vi "Cycle 9 Speed Monitor.vi"(0 "GEA2 Reference In":refnum<k24>, 5 "GEA Inputs":T1={"Source"=228, "Destination"=35} {"Destination" format="%.0x"; "Source" format="%.0x"}, 7 "Standalone?":bool, 11 "Error In":errorcluster) -> (4 "GEA2 Reference Out":refnum<k24>, 6 "Pass/Fail?":bool, 8 "Report Text":string, 15 "Error Out":errorcluster)   [LabVIEW 2016, in "Centauro.lvlib"]
uses:
  Projects/Centauro.lvlib
  Q:/Common/DLLs/GEA3/GeaCommunication.dll
  Common/DLLs/GEA3/GeaCommunication.dll
  Common/LabVIEW GEA2 Toolkit/LabVIEW_GEA2_Toolkit.lvlibp/type defs/Source_Destination.ctl
  Common/LabVIEW GEA2 Toolkit/LabVIEW_GEA2_Toolkit.lvlibp/type defs/ERD Read Data In.ctl
  Common/LabVIEW GEA2 Toolkit/LabVIEW_GEA2_Toolkit.lvlibp/type defs/Data Type.ctl
  Valew Common/type defs/Drive Cycle Engine Request State.ctl
  Common/LabVIEW GEA2 Toolkit/LabVIEW_GEA2_Toolkit.lvlibp
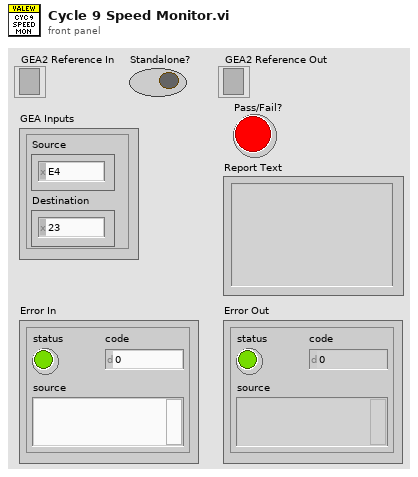
[diagram p1: front panel]
types:
  T1 = typedef "LabVIEW_GEA2_Toolkit.lvlibp/Source_Destination.ctl" = cluster{"Source":u8, "Destination":u8}
  T2 = typedef "LabVIEW_GEA2_Toolkit.lvlibp/ERD Read Data In.ctl" = cluster{"ERD Number":u16, "Data Type":T3}
  T3 = typedef "LabVIEW_GEA2_Toolkit.lvlibp/Data Type.ctl" = enum16{"string", "boolean", "uint8_t", "uint16_t", "uint32_t", "uint64_t", "int8_t", "int16_t", "int32_t", "int64_t"}
  T4 = enum16{"EQ (==)", "NE (!=)", "GT (>)", "LT (<)", "GE (>=)", "LE (<=)", "GTLT(> <)", "GELE (>= <=)", "GELT (>= <)", "GTLE (> <=)", "LTGT (< >)", "LEGE (<= >=)", "LEGT (<= >)", "LTGE (< >=)", "No Comparison"}
  T5 = typedef "Centauro.lvlib/Drive Cycle Engine Request State.ctl" = enum16{"Start", "Stop", "Pause", "Resume", "Select"}
  T6 = typedef "LabVIEW_GEA2_Toolkit.lvlibp/ERD Read Data Out.ctl" = cluster{"ERD Number":u16, "Data":string}
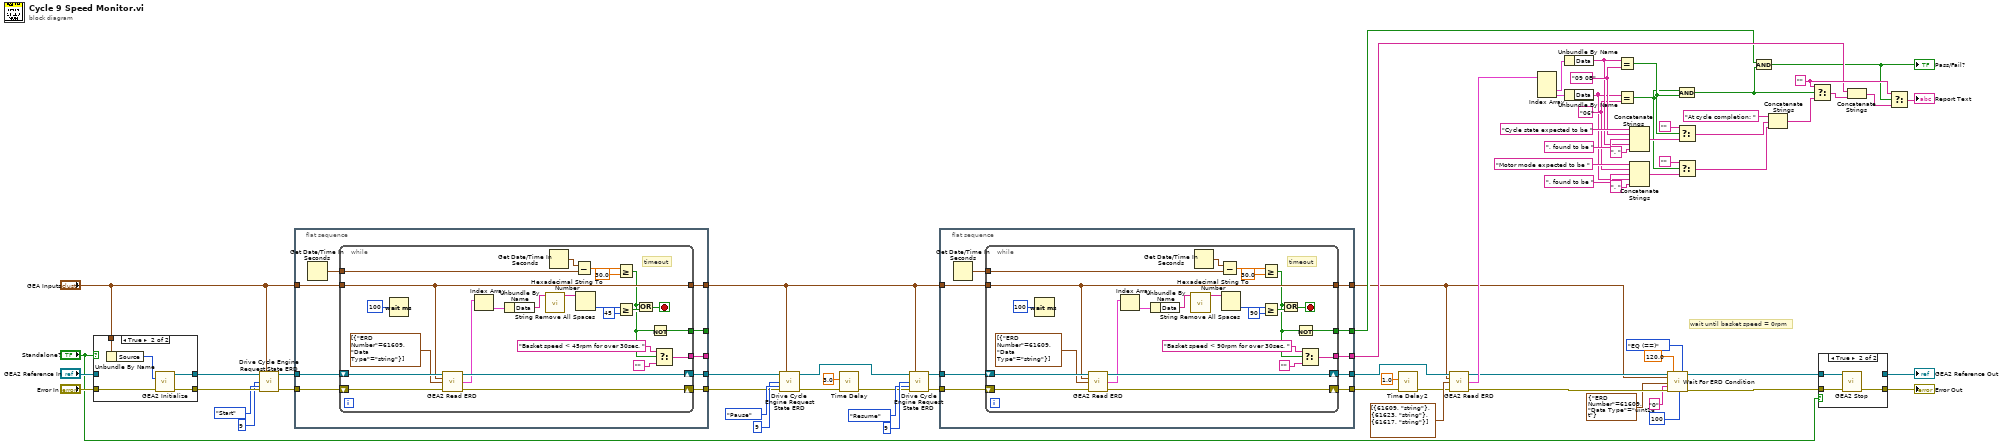
[diagram p0: block diagram]
diagram:
  w30 = ""
  w66 = "09 0B" ("y")
  w54 = "06" ("y")
  # "wait until basket speed = 0rpm"
  n1 = case shown="True" "Standalone?" {
    tunnel: "GEA2 Reference In" -> [w73 _]
    tunnel: [w73 w78] -> w34
    tunnel: "Error In" -> [w72 w77]
    tunnel: [w72 w76] -> w33
    tunnel: "GEA Inputs" -> [_ w75]
    frame False {
    }
    frame True {
      n2 = Unbundle By Name(w75) -> ("Source"=w74:u8)
      n3 = call "GEA2 Initialize.vi"("Source Address"=w74, "error in"=w77) -> ("GEA2 Reference Out"=w78:refnum<k24>, "error out"=w76:errorcluster)  [unwired: 11 in, 1 out]
    }
  }
  n4 = call "Drive Cycle Engine Request State ERD.vi"("GEA2 Reference In"=w34, "GEA Inputs"="GEA Inputs", "Cycle ID"=u8 9, "Drive Cycle Engine Request State"=Drive_Cycle_Engine_Request_State."Start", "Error In"=w33) -> ("GEA2 Reference Out"=w20:refnum<k24>, "Error Out"=w19:errorcluster)  [unwired: 9 in]
  n5 = flat-sequence {
    tunnel: [w84] -> w17
    tunnel: [w83] -> w18
    tunnel: [w82] -> w16
    tunnel: [w80] -> _
    tunnel: [w81] -> _
    tunnel: w19 -> [w85]
    tunnel: "GEA Inputs" -> [w86]
    tunnel: w20 -> [w87]
    frame #0 {
      n6 = Get Date/Time In Seconds() -> (seconds since 1Jan1904=w79:timestamp)
      n7 = while {
        shift-right: [w110] -> w84
        shift-left: w85 -> [w111]
        shift-right: [w108] -> w83
        shift-left: w87 -> [w109]
        tunnel: w86 -> [w106]
        tunnel: [w106] -> w82
        tunnel: w79 -> [w89]
        tunnel: [w92] -> w81
        tunnel: [w90] -> w80
        stop <- w103 stop-if-true
        # "timeout"
        n8 = Wait (ms)(milliseconds to wait=u32 100) -> ()  [unwired: 1 out]
        n9 = call "GEA2 Read ERD.vi"("GEA2 Reference In"=w109, "GEA Inputs"=w106, "Read ERD List"=T2[] [{"ERD Number"=61609, "Data Type"=enum."string"}], "Error In"=w111) -> ("GEA2 Reference Out"=w108:refnum<k24>, "ERD Data Out"=w96:T6[], "Error Out"=w110:errorcluster)  [unwired: 8 in, 1 out]
        n10 = Index Array(array=w96) -> (element=w107:T6)  [unwired: 1 in]
        n11 = Unbundle By Name(w107) -> ("Data"=w99:string)
        n12 = call "String Remove All Spaces.vi"("Input String"=w99) -> ("Spaces Removed"=w100:string)  [unwired: 13 in, 1 out]
        n13 = Get Date/Time In Seconds() -> (seconds since 1Jan1904=w104:timestamp)
        n14 = Subtract(x=w104, y=w89) -> (x-y=w105:dbl)
        n15 = Hexadecimal String To Number(string=w100) -> (number=w98:u32)  [unwired: 2 in, 1 out]
        n16 = Greater Or Equal?(x=w105, y=30.0) -> (x >= y?=w91:bool)
        n17 = Greater Or Equal?(x=w98, y=u32 45) -> (x >= y?=w95:bool)
        n18 = Or(x=w91, y=w95) -> (x .or. y?=w103:bool)
        n19 = Not(x=w91) -> (.not. x?=w90:bool)
        n20 = Select(t="Basket speed < 45rpm for over 30sec. ", s=w91, f="") -> (s? t:f=w92:string)
      }
    }
  }
  n21 = call "Drive Cycle Engine Request State ERD.vi"("GEA2 Reference In"=w18, "GEA Inputs"=w16, "Cycle ID"=u8 9, "Drive Cycle Engine Request State"=Drive_Cycle_Engine_Request_State."Pause", "Error In"=w17) -> ("GEA2 Reference Out"=w36:refnum<k24>, "Error Out"=w40:errorcluster)  [unwired: 9 in]
  n22 = call "Time Delay"("error in (no error)"=w40, "Delay Time (s)"=3.0) -> ("error out"=w37:errorcluster)  [unwired: 9 in]
  n23 = call "Drive Cycle Engine Request State ERD.vi"("GEA2 Reference In"=w36, "GEA Inputs"=w16, "Cycle ID"=u8 9, "Drive Cycle Engine Request State"=Drive_Cycle_Engine_Request_State."Resume", "Error In"=w37) -> ("GEA2 Reference Out"=w25:refnum<k24>, "Error Out"=w14:errorcluster)  [unwired: 9 in]
  n24 = flat-sequence {
    tunnel: [w117] -> w12
    tunnel: [w116] -> w24
    tunnel: [w115] -> w4
    tunnel: [w113] -> w22
    tunnel: [w114] -> w23
    tunnel: w14 -> [w118]
    tunnel: w16 -> [w119]
    tunnel: w25 -> [w120]
    frame #0 {
      n25 = Get Date/Time In Seconds() -> (seconds since 1Jan1904=w112:timestamp)
      n26 = while {
        shift-right: [w143] -> w117
        shift-left: w118 -> [w144]
        shift-right: [w141] -> w116
        shift-left: w120 -> [w142]
        tunnel: w119 -> [w139]
        tunnel: [w139] -> w115
        tunnel: w112 -> [w122]
        tunnel: [w125] -> w114
        tunnel: [w123] -> w113
        stop <- w136 stop-if-true
        # "timeout"
        n27 = Wait (ms)(milliseconds to wait=u32 100) -> ()  [unwired: 1 out]
        n28 = call "GEA2 Read ERD.vi"("GEA2 Reference In"=w142, "GEA Inputs"=w139, "Read ERD List"=T2[] [{"ERD Number"=61609, "Data Type"=enum."string"}], "Error In"=w144) -> ("GEA2 Reference Out"=w141:refnum<k24>, "ERD Data Out"=w129:T6[], "Error Out"=w143:errorcluster)  [unwired: 8 in, 1 out]
        n29 = Index Array(array=w129) -> (element=w140:T6)  [unwired: 1 in]
        n30 = Unbundle By Name(w140) -> ("Data"=w132:string)
        n31 = call "String Remove All Spaces.vi"("Input String"=w132) -> ("Spaces Removed"=w133:string)  [unwired: 13 in, 1 out]
        n32 = Get Date/Time In Seconds() -> (seconds since 1Jan1904=w137:timestamp)
        n33 = Subtract(x=w137, y=w122) -> (x-y=w138:dbl)
        n34 = Hexadecimal String To Number(string=w133) -> (number=w131:u32)  [unwired: 2 in, 1 out]
        n35 = Greater Or Equal?(x=w138, y=30.0) -> (x >= y?=w124:bool)
        n36 = Greater Or Equal?(x=w131, y=u32 90) -> (x >= y?=w128:bool)
        n37 = Or(x=w124, y=w128) -> (x .or. y?=w136:bool)
        n38 = Not(x=w124) -> (.not. x?=w123:bool)
        n39 = Select(t="Basket speed < 90rpm for over 30sec. ", s=w124, f="") -> (s? t:f=w125:string)
      }
    }
  }
  n40 = call "Time Delay2"("error in (no error)"=w12, "Delay Time (s)"=1.0) -> ("error out"=w13:errorcluster)  [unwired: 9 in]
  n41 = call "GEA2 Read ERD.vi"("GEA2 Reference In"=w24, "GEA Inputs"=w4, "Read ERD List"=T2[] [{"ERD Number"=61609, "Data Type"=enum."string"}, {"ERD Number"=61623, "Data Type"=enum."string"}, {"ERD Number"=61617, "Data Type"=enum."string"}], "Error In"=w13) -> ("GEA2 Reference Out"=w10:refnum<k24>, "ERD Data Out"=w68:T6[], "Error Out"=w9:errorcluster)  [unwired: 8 in, 1 out]
  n42 = Index Array(array=w68) -> (element #2=w71:T6, element #3=w70:T6)  [unwired: 3 in, 1 out]
  n43 = Unbundle By Name(w71) -> ("Data"=w64:string)
  n44 = Unbundle By Name(w70) -> ("Data"=w52:string)
  n45 = Equal?(x=w64, y=w66) -> (x = y?=w61:bool)
  n46 = Equal?(x=w52, y=w54) -> (x = y?=w60:bool)
  n47 = Concatenate Strings("Cycle state expected to be " ("string"), w66, ", found to be " ("string"), w64, ". " ("string")) -> (w62:string)
  n48 = Concatenate Strings("Motor mode expected to be " ("string"), w54, ", found to be " ("string"), w52, ". " ("string")) -> (w57:string)
  n49 = call "Wait For ERD Condition.vi"("GEA2 Reference In"=w10, "GEA Inputs"=w4, "ERD Read Data"=T2 {"ERD Number"=61609, "Data Type"=enum."uint16_t"}, "Expected Low"="0", "Error In"=w9, "Timeout (s)"=120.0, "Loop Rate (ms)"=u32 100, "Comparison"=T4."EQ (==)") -> ("GEA2 Reference Out"=w6:refnum<k24>, "Error Out"=w5:errorcluster)  [unwired: 7 in, 3 out]
  n50 = And(x=w60, y=w61) -> (x .and. y?=w32:bool)
  n51 = Select(t="", s=w61, f=w62) -> (s? t:f=w50:string)
  n52 = Select(t="", s=w60, f=w57) -> (s? t:f=w49:string)
  n53 = And(x=w22, y=w32) -> (x .and. y?=w21:bool)
  "Pass/Fail?" <- w21
  n54 = Concatenate Strings("At cycle completion: " ("string"), w50, w49) -> (w56:string)
  n55 = Select(t=w30, s=w32, f=w56) -> (s? t:f=w31:string)
  n56 = case shown="True" "Standalone?" {
    tunnel: [w145 w149] -> w45
    tunnel: w5 -> [w145 w148]
    tunnel: w6 -> [w146 w147]
    tunnel: [w146 _] -> w43
    frame False {
    }
    frame True {
      n57 = call "GEA2 Stop.vi"("GEA2 Reference In"=w147, "Error In"=w148) -> ("Error Out"=w149:errorcluster)  [unwired: 13 in]
    }
  }
  "GEA2 Reference Out" <- w43
  "Error Out" <- w45
  n58 = Concatenate Strings(w23, w31) -> (w29:string)
  n59 = Select(t=w30, s=w21, f=w29) -> (s? t:f=→"Report Text":string)
